vi "get_raw_data.vi"() -> ()   [LabVIEW 2017]
uses:
  <vilib>/Utility/file.llb/Read Delimited Spreadsheet (I64).vi
panel:
  out "coarse_counter1":u64=65198835 format="%x"
  out "coarse_counter2":u64=65198835 format="%x"
  out "fine2":u64 format="%x"
  out "fine1":u64 format="%x"
  out "coarse2":u64
  out "coarse1":u64
  out "raw2":u64=65198835 format="%x"
  out "raw1":u64=65198835 format="%x"
  in  "index (row) 2":i32
  in  "index (row)":i32
  in  "file path (dialog if empty)":path
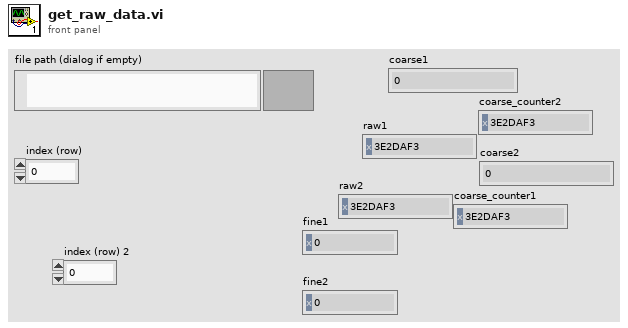
[diagram p1: front panel]
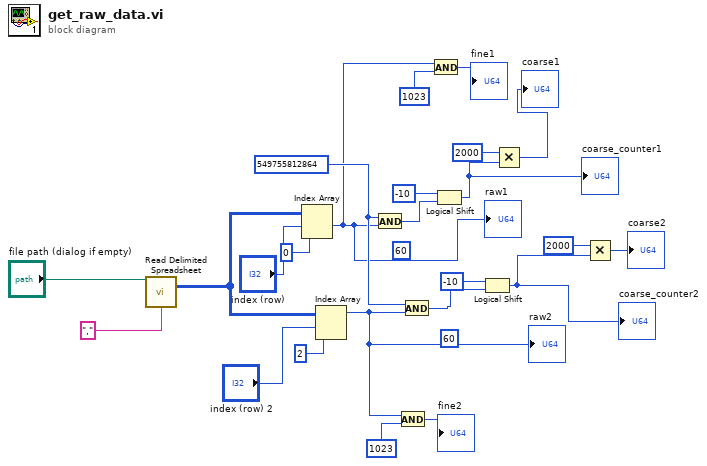
[diagram p0: block diagram]
diagram:
  (unwired) u64 60 ("x")
  w13 = u64 549755812864 ("port")
  (unwired) u64 60 ("x")
  n1 = call-poly <vilib>:"Read Delimited Spreadsheet.vi"("file path (dialog if empty)"="file path (dialog if empty)", "delimiter (\\t)"="," ("delimiter (\\t)")) -> ("all rows"=w18:i64[][])  [unwired: 8 in, 5 out]
  n2 = Index Array(array=w18, index (row)="index (row)", index (col)=0 ("disabled index (col)")) -> (element=w4:i64)
  "raw1" <- w4
  n3 = Index Array(array=w18, index (row)="index (row) 2", index (col)=2 ("disabled index (col)")) -> (element=w3:i64)
  "raw2" <- w3
  n4 = And(x=w13, y=w4) -> (x .and. y?=w16:u64)
  n5 = And(x=w3, y=u64 1023 ("port")) -> (x .and. y?=→"fine2":u64)
  n6 = And(x=w13, y=w3) -> (x .and. y?=w14:u64)
  n7 = And(x=w4, y=u64 1023 ("port")) -> (x .and. y?=→"fine1":u64)
  n8 = Logical Shift(y=i16 -10, x=w16) -> (x << y=w1:u64)
  "coarse_counter1" <- w1
  n9 = Logical Shift(y=i16 -10, x=w14) -> (x << y=w2:u64)
  "coarse_counter2" <- w2
  n10 = Multiply(x=u64 2000, y=w1) -> (x*y=→"coarse1":u64)
  n11 = Multiply(x=u64 2000, y=w2) -> (x*y=→"coarse2":u64)
